vi "Write_Wrap.vi"(8 "error in (no error)":errorcluster, 10 "Value":T1, 11 "Var_DBL in":refnum<class "Var_U8.lvclass">) -> (0 "error out":errorcluster, 3 "Var_DBL out":refnum<class "Var_U8.lvclass">)   [LabVIEW 2021, in "Var_U8.lvclass"]
uses:
  Var_U8.lvclass
  Type.ctl
  Var_U8.lvclass/Var_U8.ctl
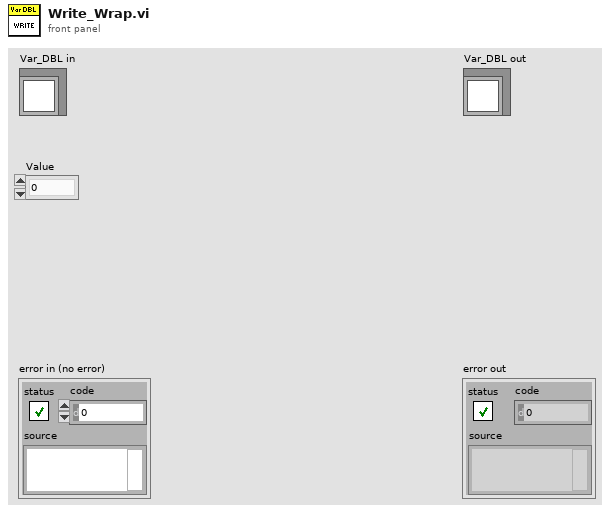
[diagram p1: front panel]
types:
  T1 = typedef "Var_U8.lvclass/Type.ctl" = dbl
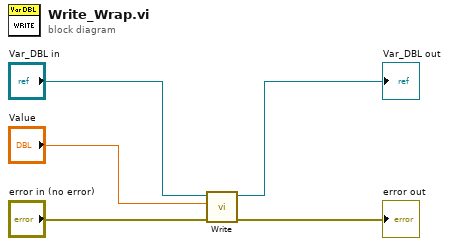
[diagram p0: block diagram]
diagram:
  n1 = call-dynamic "Write.vi"("error in (no error)"="error in (no error)", "Value"="Value", "Double Float.lvclass_340760 in"="Var_DBL in") -> ("error out"=→"error out":errorcluster, "Double Float.lvclass_340760 out"=→"Var_DBL out":refnum<class "Var_U8.lvclass">)  [unwired: 7 in]
